vi "RNDPowerSupplyGUI_logger.vi"() -> ()   [LabVIEW 2011]
panel:
  in  "Path":path=path "C:/temp/RNDPower.log"
  in  "On":bool=TRUE
  out "Watt":dbl
  out "Ohm":dbl
  out "error out":errorcluster
  in  "Port 7?":refnum<visa-resource-name>
  in  "Update rate [s]":dbl=3.0 min=1.0 max=100.0 step=0.1
  in  "stop":bool
  out "Waveform Chart":dbl[][](graph)
  in  "Ampere":dbl(knob) scale=0.0..5.0
  in  "Volt":dbl(knob) scale=0.0..20.0 scale format="%#_3g"
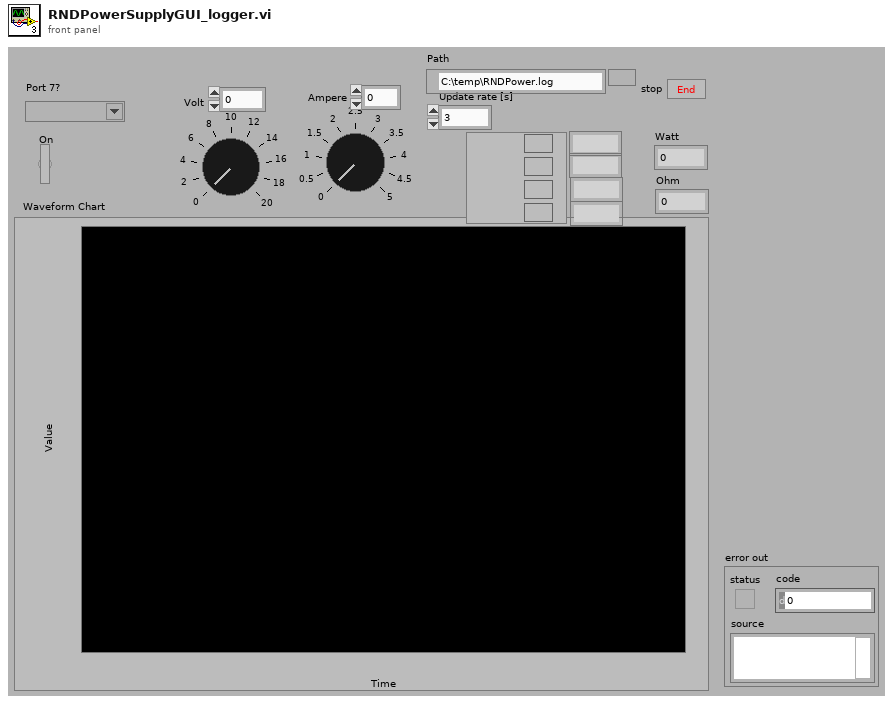
[diagram p1: front panel]
types:
  T1 = enum16{"open", "replace", "create", "open or create", "replace or create", "replace or create with confirmation"}
  T2 = enum16{"No Operation", "GetActualUI", "GetSetpointsUI", "SetUI", "SetU", "SetI", "OutputOff", "OutputOn", "GetLimitU", "GetLimitI", "SetLimitU", "SetLimitI", "GetUI-fromVersion", "RawCommand"}
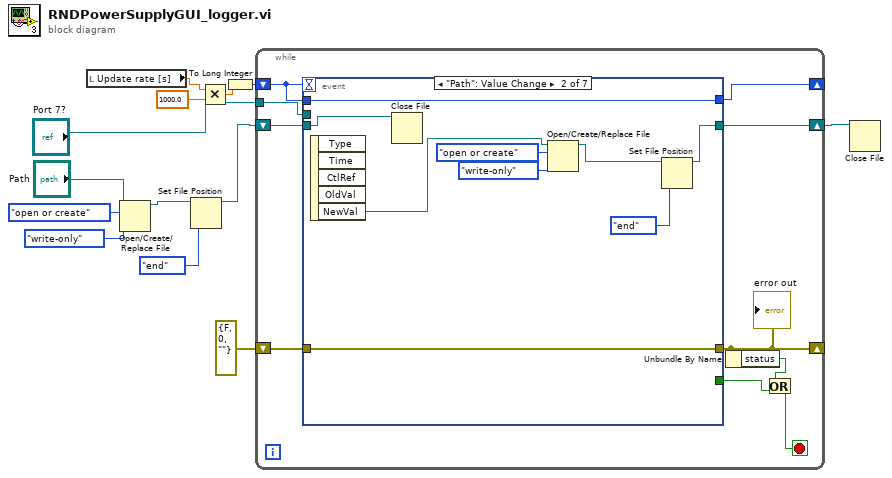
[diagram p0: block diagram]
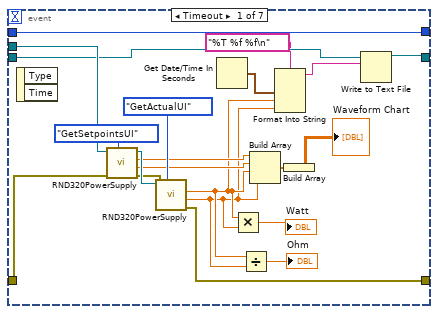
[diagram p2: hidden frame]
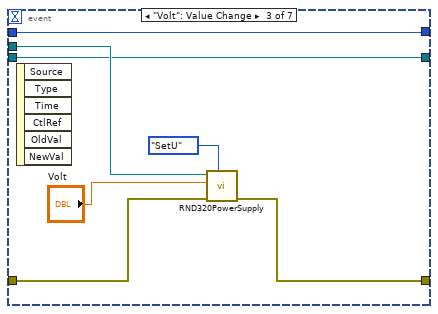
[diagram p3: hidden frame]
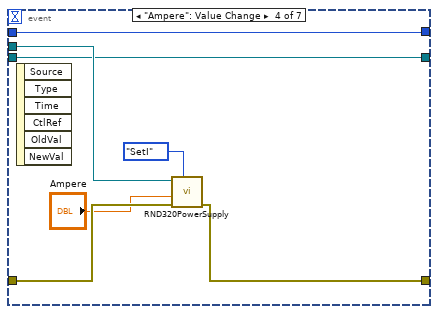
[diagram p4: hidden frame]
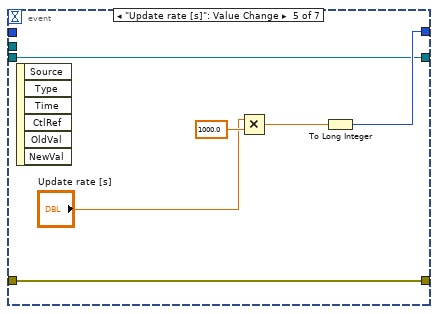
[diagram p5: hidden frame]
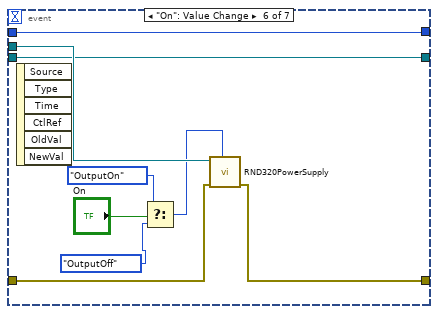
[diagram p6: hidden frame]
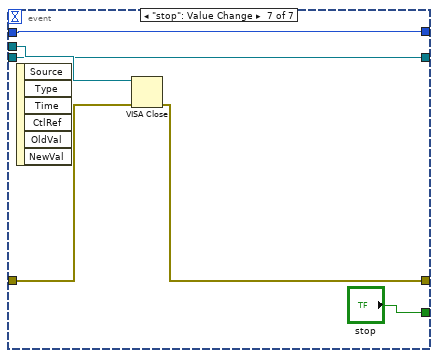
[diagram p7: hidden frame]
diagram:
  n1 = local read "Update rate [s]"() -> (w13:dbl)
  n2 = Open/Create/Replace File(file path (use dialog)="Path", operation (0:open)=T1."open or create", access (0:read/write)=enum16{"read/write", "read-only", "write-only"}."write-only") -> (refnum out=w3:refnum<file>)  [unwired: 3 in, 2 out]
  n3 = Set File Position(refnum=w3, from (0:start)=enum16{"start", "end", "current"}."end") -> (refnum out=w2:refnum<file>)  [unwired: 2 in, 1 out]
  n4 = Multiply(x=w13, y=1000.0) -> (x*y=w11:dbl)
  n5 = To Long Integer(number=w11) -> (32bit integer=w10:i32)
  n6 = while {
    shift-right: [w23] -> _
    shift-left: w10 -> [w20]
    tunnel: "Port 7?" -> [w22]
    shift-right: [w19] -> _
    shift-left: errorcluster {"status"=FALSE, "code"=0, "source"=""} ("error out") -> [w21]
    shift-right: [w15] -> w6
    shift-left: w2 -> [w14]
    stop <- w16 stop-if-true
    n7 = event shown="[1] \"Path\": Value Change" {
      selector: _ -> [_ _ _ _ _ _ _]
      dyn-events: _ -> [_ _ _ _ _ _ _]
      timeout: w20 -> [_ _ _ _ _ _ _]
      tunnel: [_ _ _ _ _ _ "stop"] -> w18
      tunnel: [w34 w49 w56 w63 w70 w75 w86] -> w23
      tunnel: w22 -> [w44 _ w55 w62 _ w82 w87]
      tunnel: [w38 w48 w60 w66 w69 w76 w84] -> w19
      tunnel: w21 -> [w40 w48 w59 w67 w69 w77 w85]
      tunnel: w20 -> [w34 w49 w56 w63 _ w75 w86]
      tunnel: [w31 w45 w54 w61 w68 w74 w83] -> w15
      tunnel: w14 -> [w30 w53 w54 w61 w68 w74 w83]
      event Timeout {
        n8 = event-data() -> ()  [unwired: 3 out]
        n9 = call "RND320PowerSupply.vi"("Command"=T2."GetSetpointsUI", "error in (no error)"=w40, "VISA resource name"=w44) -> ("error out"=w39:errorcluster, "Ampere out"=w36:dbl, "Volt out"=w37:dbl, "VISA resource name out"=w43:refnum<visa-resource-name>)  [unwired: 4 in, 1 out]
        n10 = call "RND320PowerSupply.vi"("Command"=T2."GetActualUI", "error in (no error)"=w39, "VISA resource name"=w43) -> ("error out"=w38:errorcluster, "Ampere out"=w27:dbl, "Volt out"=w28:dbl)  [unwired: 4 in, 2 out]
        n11 = Get Date/Time In Seconds() -> (seconds since 1Jan1904=w26:timestamp)
        n12 = Multiply(x=w28, y=w27) -> (x*y=→"Watt":dbl)
        n13 = Divide(x=w28, y=w27) -> (x/y=→"Ohm":dbl)
        n14 = Build Array(w37, w36, w28, w27) -> (w29:dbl[])
        n15 = Format Into String(format string="%T %f %f\n", w26, w28, w27) -> (resulting string=w24:string)  [unwired: 2 in, 1 out]
        n16 = Build Array(w29) -> (→"Waveform Chart":dbl[][])
        n17 = Write to Text File(file (use dialog)=w30, text=w24) -> (refnum out=w31:refnum<file>)  [unwired: 2 in, 2 out]
      }
      event "Path": Value Change {
        n18 = event-data() -> ("NewVal"=w50:path)  [unwired: 5 out]
        n19 = Close File(refnum=w53) -> ()  [unwired: 1 in, 2 out]
        n20 = Open/Create/Replace File(file path (use dialog)=w50, operation (0:open)=T1."open or create", access (0:read/write)=enum16{"read/write", "read-only", "write-only"}."write-only") -> (refnum out=w46:refnum<file>)  [unwired: 3 in, 2 out]
        n21 = Set File Position(refnum=w46, from (0:start)=enum16{"start", "end", "current"}."end") -> (refnum out=w45:refnum<file>)  [unwired: 2 in, 1 out]
      }
      event "Volt": Value Change {
        n22 = event-data() -> ()  [unwired: 7 out]
        n23 = call "RND320PowerSupply.vi"("Command"=T2."SetU" ("Enum"), "error in (no error)"=w59, "Volt in"="Volt", "VISA resource name"=w55) -> ("error out"=w60:errorcluster)  [unwired: 3 in, 4 out]
      }
      event "Ampere": Value Change {
        n24 = event-data() -> ()  [unwired: 7 out]
        n25 = call "RND320PowerSupply.vi"("Command"=T2."SetI" ("Enum"), "error in (no error)"=w67, "Ampere"="Ampere", "VISA resource name"=w62) -> ("error out"=w66:errorcluster)  [unwired: 3 in, 4 out]
      }
      event "Update rate [s]": Value Change {
        n26 = event-data() -> ()  [unwired: 7 out]
        n27 = Multiply(x="Update rate [s]", y=1000.0) -> (x*y=w71:dbl)
        n28 = To Long Integer(number=w71) -> (32bit integer=w70:i32)
      }
      event "On": Value Change {
        n29 = event-data() -> ()  [unwired: 7 out]
        n30 = Select(t=T2."OutputOn" ("Enum"), s="On", f=T2."OutputOff" ("Enum")) -> (s? t:f=w78:T2)
        n31 = call "RND320PowerSupply.vi"("Command"=w78, "error in (no error)"=w77, "VISA resource name"=w82) -> ("error out"=w76:errorcluster)  [unwired: 4 in, 4 out]
      }
      event "stop": Value Change {
        n32 = event-data() -> ()  [unwired: 7 out]
        n33 = VISA Close(VISA resource name=w87, error in (no error)=w85) -> (error out=w84:errorcluster)
      }
    }
    "error out" <- w19
    n34 = Unbundle By Name(w19) -> ("status"=w17:bool)
    n35 = Or(x=w17, y=w18) -> (x .or. y?=w16:bool)
  }
  n36 = Close File(refnum=w6) -> ()  [unwired: 1 in, 2 out]
